vi "InsertNewItem.vi"(7 "Replace?":bool, 8 "error in (no error)":errorcluster, 9 "ILabVIEWItem in":refnum<class "ILabVIEWItem.lvclass">, 11 "CDependencyList in":refnum<class "CDependencyList.lvclass">) -> (0 "error out":errorcluster, 2 "New key?":bool, 3 "CDependencyList out":refnum<class "CDependencyList.lvclass">)   [LabVIEW 2020, in "DependencyInspection.lvlib" / "CDependencyList.lvclass"]
uses:
  CDependencyList.lvclass
  <vilib>/Utility/miscctls.llb/LVMapReplaceAction.ctl
  LabVIEWObjectInterfaces/ILabVIEWItem/ILabVIEWItem.lvclass
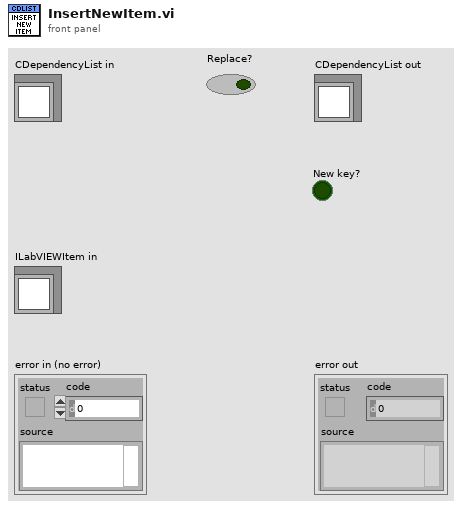
[diagram p1: front panel]
types:
  T1 = typedef "LVMapReplaceAction.ctl" = enum32{"Modify Entry only if found", "Add or Modify Entry", "Delete Entry"}
  T2 = typedef "DependencyInspection.lvlib/CDependencyList.lvclass/DependencyListRef.ctl" = refnum<data-value>
  T3 = typedef "DependencyInspection.lvlib/CDependencyList.lvclass/DependencyList.ctl" = map{string, refnum<class "ILabVIEWItem.lvclass">}
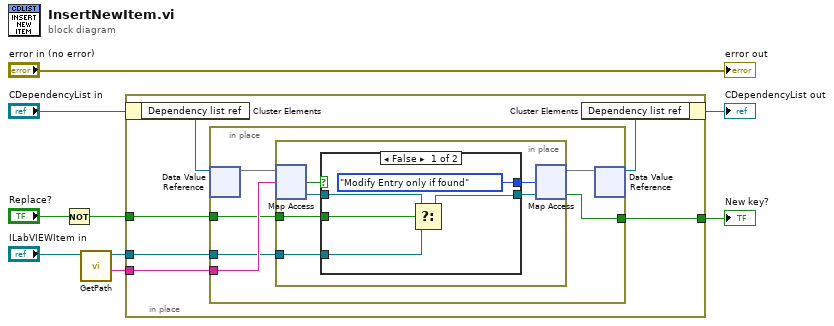
[diagram p0: block diagram]
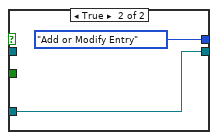
[diagram p2: hidden frame]
diagram:
  n1 = Not(x="Replace?") -> (.not. x?=w3:bool)
  n2 = call-dynamic "GetPath.vi"("ILabVIEWItem in"="ILabVIEWItem in") -> ("Path"=w8:string, "ILabVIEWItem out"=w7:refnum<class "ILabVIEWItem.lvclass">)  [unwired: 8 in, 1 out]
  n3 = in-place {
    in-place-border: w8 -> [w15]
    in-place-border: w7 -> [w14]
    in-place-border: [w13] -> w5
    in-place-border: w3 -> [w12]
    n4 = in-place-cluster #1("CDependencyList in") -> ("Dependency list ref"=w11:T2)
    n5 = in-place {
      in-place-border: w15 -> [w21]
      in-place-border: w14 -> [w20]
      in-place-border: [w19] -> w13
      in-place-border: w12 -> [w18]
      n6 = in-place-dvr #2(w11) -> (w17:T3)  [unwired: 1 out]
      n7 = in-place {
        in-place-border: w20 -> [w23]
        in-place-border: w18 -> [w22]
        n8 = in-place-map #3(w17, w21) -> (w24:refnum<class "ILabVIEWItem.lvclass">, w27:bool)  [unwired: 1 in]
        n9 = case shown="False" w27 {
          tunnel: [LVMapReplaceAction."Modify Entry only if found" ("action") LVMapReplaceAction."Add or Modify Entry" ("action")] -> w26
          tunnel: [w29 w33] -> w25
          tunnel: w24 -> [w30 _]
          tunnel: w23 -> [w28 w33]
          tunnel: w22 -> [w31 _]
          frame False {
            n10 = Select(t=w30, s=w31, f=w28) -> (s? t:f=w29:refnum<class "ILabVIEWItem.lvclass">)
          }
          frame True {
          }
        }
        n11 = in-place-map #3(w25, w26) -> (w16:T3, w19:bool)  [unwired: 1 out]
      }
      n12 = in-place-dvr #2(w16) -> (w10:T2)  [unwired: 1 out]
    }
    n13 = in-place-cluster #1("Dependency list ref"=w10) -> (→"CDependencyList out":refnum<class "CDependencyList.lvclass">)
  }
  "New key?" <- w5
  "error out" <- "error in (no error)"
